vi "Main multi.vi"(11 "Args":string[](array[string])) -> (2 "Output":string, 3 "Exit Code":i32)   [LabVIEW 2021]
uses:
  <vilib>/Utility/file.llb/Write Delimited Spreadsheet (string).vi
  Add_Library.lvlib
panel:
  in  "y":u64[](array[numeric])=[1, 2, 3]
  in  "x":u64[](array[numeric])=[1, 2, 3]
  out "x+y":u64[](array[numeric])
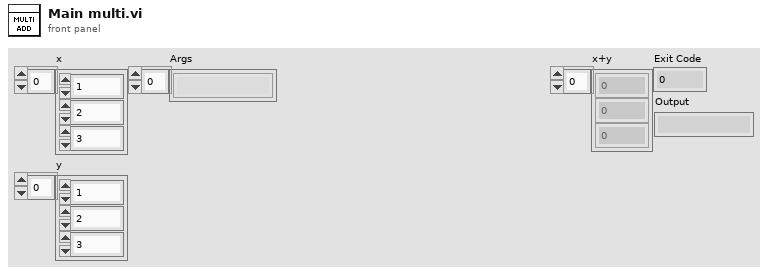
[diagram p1: front panel]
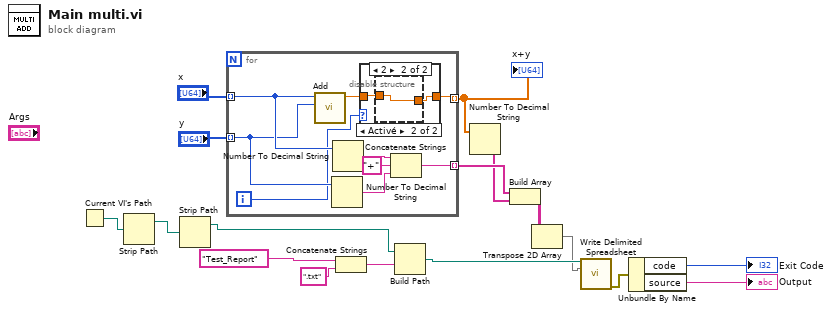
[diagram p0: block diagram]
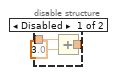
[diagram p3: hidden frame]
diagram:
  n1 = Current VI's Path() -> (path=w10:path)
  n2 = Strip Path(path=w10) -> (stripped path=w2:path)  [unwired: 1 out]
  n3 = Strip Path(path=w2) -> (stripped path=w1:path)  [unwired: 1 out]
  n4 = for {
    tunnel: "x" -> [w26] mode=indexing
    tunnel: "y" -> [w25] mode=indexing
    tunnel: [w19] -> w15 mode=indexing
    tunnel: [w21] -> w14 mode=indexing
    i -> [w18]
    n5 = call "Add.vi"("y"=w25, "x"=w26) -> ("x+y"=w20:dbl)  [unwired: 9 in]
    n6 = Number To Decimal String(number=w25) -> (decimal integer string=w22:string)  [unwired: 1 in]
    n7 = Number To Decimal String(number=w26) -> (decimal integer string=w24:string)  [unwired: 1 in]
    n8 = case shown="2" w18 {
      tunnel: w20 -> [w27 w29]
      tunnel: [w27 w28] -> w19
      frame 0, Default {
      }
      frame 2 {
        n9 = disable-structure shown="Activé" {
          disable-tunnel: w29 -> [w32 w33]
          disable-tunnel: [w30 w33] -> w28
          frame Disabled {
            n10 = Add(x=w32, y=3.0) -> (x+y=w30:dbl)
          }
          frame Enabled {
          }
        }
      }
    }
    n11 = Concatenate Strings(w24, "+" ("chaîne"), w22) -> (w21:string)
  }
  "x+y" <- w15
  n12 = Concatenate Strings("Test_Report" ("Report Path"), ".txt" ("chaîne")) -> (w9:string)
  n13 = Build Path(base path=w1, name or relative path=w9) -> (appended path=w8:path)
  n14 = Number To Decimal String(number=w15) -> (decimal integer string=w13:string[])  [unwired: 1 in]
  n15 = Build Array(w14, w13) -> (w7:string[][])
  n16 = Transpose 2D Array(2D array=w7) -> (transposed array=w6:string[][])
  n17 = call-poly <vilib>:"Write Delimited Spreadsheet.vi"("file path (dialog if empty)"=w8, "2D data"=w6) -> ("error out"=w3:errorcluster)  [unwired: 12 in, 1 out]
  n18 = Unbundle By Name(w3) -> ("code"=→"Exit Code":i32, "source"=→"Output":string)
